vi "sub Set StartTimeStamp.vi"(8 "error in (no error)":errorcluster, 10 "Start Time Stamp":timestamp, 11 "Waveform Array in":waveform(dbl)[](array[waveform])) -> (0 "error out (no error)":errorcluster, 3 "Waveform Array out":waveform(dbl)[](array[waveform]))   [LabVIEW 2017, in "Set DDT Attributes.lvlib"]
uses:
  <vilib>/express/express signal manip/GetorSetDDTAttributes/Set DDT Attributes/Set DDT Attributes.lvlib
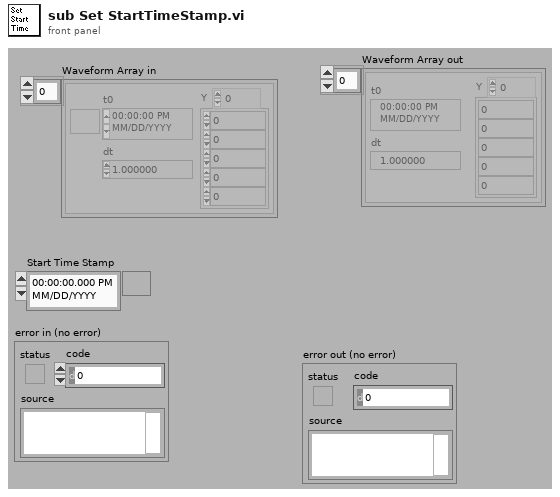
[diagram p1: front panel]
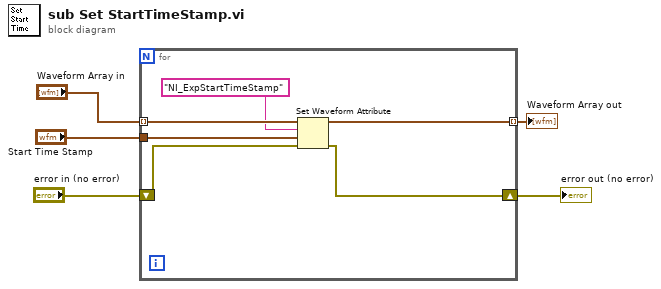
[diagram p0: block diagram]
diagram:
  n1 = for {
    tunnel: [w11] -> w1 mode=indexing
    tunnel: "Waveform Array in" -> [w10] mode=indexing
    tunnel: "Start Time Stamp" -> [w8]
    shift-right: [w6] -> w2
    shift-left: "error in (no error)" -> [w7]
    n2 = Set Waveform Attribute(4:w7, 5:w8, 6:"NI_ExpStartTimeStamp" ("name"), 7:w10) -> (0:w6:errorcluster, 3:w11:waveform(dbl))  [unwired: 1 out]
  }
  "error out (no error)" <- w2
  "Waveform Array out" <- w1
